vi "CNTR.vi"(6 "R":bool, 7 "Load":bool, 9 "DI":u32, 10 "-":bool, 11 "+":bool) -> (0 "ED":bool, 1 "EU":bool, 2 "QD":bool, 3 "QU":bool, 4 "DO":u32)   [LabVIEW 2019, in "Counter.lvlib"]
uses:
  Counter.lvlib
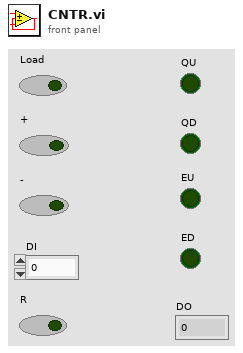
[diagram p1: front panel]
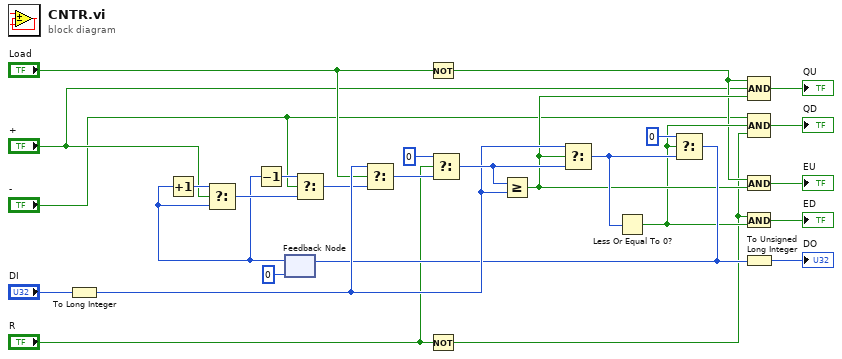
[diagram p0: block diagram]
diagram:
  n1 = To Long Integer(number="DI") -> (32bit integer=w20:i32)
  n2 = feedback #1(0) -> (w4:i32)
  n3 = Increment(x=w4) -> (x+1=w7:i32)
  n4 = Select(t=w7, s="+", f=w4) -> (s? t:f=w5:i32)
  n5 = Decrement(x=w4) -> (x-1=w6:i32)
  n6 = Select(t=w6, s="-", f=w5) -> (s? t:f=w3:i32)
  n7 = Select(t=w20, s="Load", f=w3) -> (s? t:f=w24:i32)
  n8 = Not(x="Load") -> (.not. x?=w9:bool)
  n9 = Not(x="R") -> (.not. x?=w8:bool)
  n10 = Select(t=0, s="R", f=w24) -> (s? t:f=w25:i32)
  n11 = Greater Or Equal?(x=w25, y=w20) -> (x >= y?=w13:bool)
  n12 = Select(t=w20, s=w13, f=w25) -> (s? t:f=w23:i32)
  n13 = Less Or Equal To 0?(x=w23) -> (x <= 0?=w11:bool)
  n14 = Select(t=0, s=w11, f=w23) -> (s? t:f=w18:i32)
  n15 = feedback-in #1(w18) -> ()
  n16 = And(x=w9, y=w13) -> (x .and. y?=→"EU":bool)
  n17 = And(x=w8, y=w11) -> (x .and. y?=→"ED":bool)
  n18 = To Unsigned Long Integer(number=w18) -> (unsigned 32bit integer=→"DO":u32)
  n19 = Compound Arithmetic op=AND(w9, "+", w13) -> (→"QU":bool)
  n20 = Compound Arithmetic op=AND("-", w11, w8) -> (→"QD":bool)
